vi "Cents2DollarString.vi"(10 "Cents":dbl) -> (2 "Dollars":string)   [LabVIEW 2019]
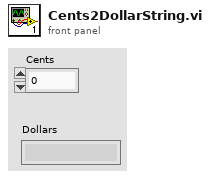
[diagram p1: front panel]
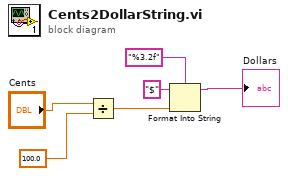
[diagram p0: block diagram]
diagram:
  n1 = Divide(x="Cents", y=100.0) -> (x/y=w4:dbl)
  n2 = Format Into String(format string="%3.2f", initial string="$", w4) -> (resulting string=→"Dollars":string)  [unwired: 1 in, 1 out]
